vi "ImPro - Sharpen.vi"(8 "error in (no error)":errorcluster, 10 "24-bit pixmap In":u32[][](array[numeric]), 11 "Sharpen?":bool) -> (0 "error out":errorcluster, 2 "24-bit pixmap Out":u32[][](array[numeric]))   [LabVIEW 2023]
panel:
  in  "Scaling Factor":dbl=5.0 min=0.0
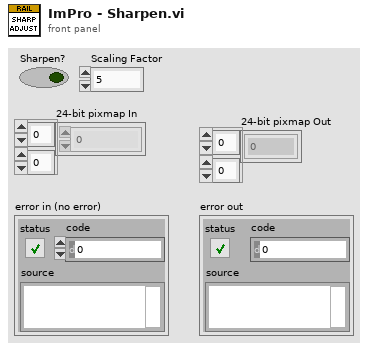
[diagram p1: front panel]
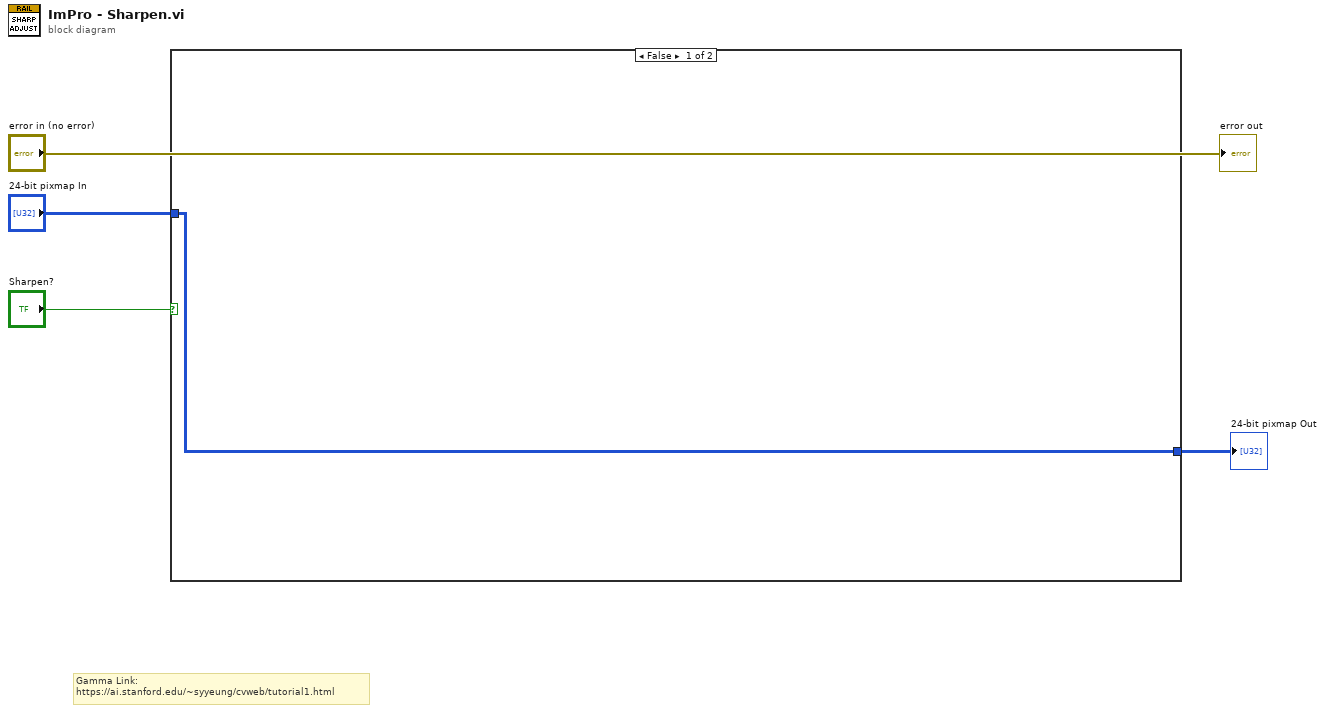
[diagram p0: block diagram]
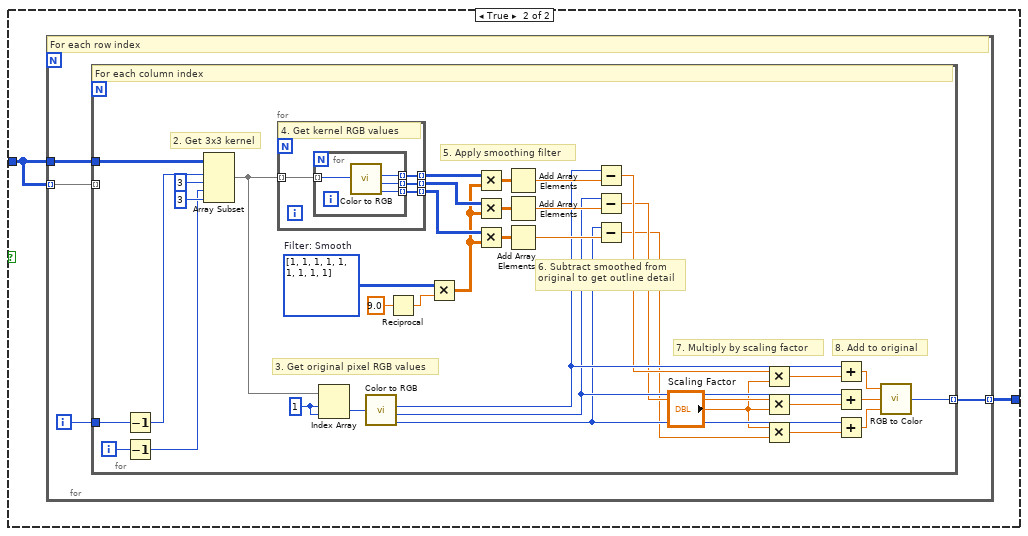
[diagram p2: hidden frame]
diagram:
  # "Gamma Link:\nhttps://ai.stanford.edu/~syyeung/cvweb/tutorial1.html"
  n1 = case shown="False" "Sharpen?" {
    tunnel: "24-bit pixmap In" -> [w5 w7]
    tunnel: [w5 w6] -> w2
    frame False {
    }
    frame True {
      n2 = for {
        tunnel: w7 -> [w11] mode=indexing
        tunnel: w7 -> [w10]
        tunnel: [w8] -> w6 mode=indexing
        i -> [w9]
        # "For each row index"
        n3 = for {
          tunnel: w11 -> [_] mode=indexing
          tunnel: w9 -> [w45]
          tunnel: w10 -> [w47]
          tunnel: [w35] -> w8 mode=indexing
          i -> [w44]
          w29 = 1 ("index (row)")
          w33 = i32[][] [[1, 1, 1], [1, 1, 1], [1, 1, 1]]  # Filter: Smooth
          # "8. Add to original"
          # "7. Multiply by scaling factor"
          # "6. Subtract smoothed from\noriginal to get outline detail"
          # "5. Apply smoothing filter"
          # "3. Get original pixel RGB values"
          # "2. Get 3x3 kernel"
          # "For each column index"
          n4 = Decrement(x=w45) -> (x-1=w43:i32)
          n5 = Decrement(x=w44) -> (x-1=w42:i32)
          n6 = Array Subset(array=w47, index (row)=w43, length (row)=3 ("length"), index (col)=w42, length (col)=3 ("length")) -> (w30:u32[][])
          n7 = for {
            tunnel: w30 -> [w52] mode=indexing
            tunnel: [w51] -> w40 mode=indexing
            tunnel: [w50] -> w37 mode=indexing
            tunnel: [w49] -> w36 mode=indexing
            # "4. Get kernel RGB values"
            n8 = for {
              tunnel: w52 -> [w56] mode=indexing
              tunnel: [w55] -> w51 mode=indexing
              tunnel: [w54] -> w50 mode=indexing
              tunnel: [w53] -> w49 mode=indexing
              n9 = call <vilib>:"Color to RGB.vi"("Color"=w56) -> ("R"=w55:u8, "G"=w54:u8, "B"=w53:u8)  [unwired: 1 out]
            }
          }
          n10 = Index Array(array=w30, index (row)=w29, index (col)=w29) -> (element=w28:u32)
          n11 = call <vilib>:"Color to RGB.vi"("Color"=w28) -> ("R"=w24:u8, "G"=w23:u8, "B"=w22:u8)  [unwired: 1 out]
          n12 = Reciprocal(x=9.0) -> (1/x=w34:dbl)
          n13 = Multiply(x=w33, y=w34) -> (x*y=w31:dbl[][])
          n14 = Multiply(x=w40, y=w31) -> (x*y=w41:dbl[][])
          n15 = Multiply(x=w37, y=w31) -> (x*y=w39:dbl[][])
          n16 = Multiply(x=w36, y=w31) -> (x*y=w38:dbl[][])
          n17 = Add Array Elements(numeric array=w41) -> (sum=w27:dbl)
          n18 = Add Array Elements(numeric array=w39) -> (sum=w25:dbl)
          n19 = Add Array Elements(numeric array=w38) -> (sum=w26:dbl)
          n20 = Subtract(x=w24, y=w27) -> (x-y=w17:dbl)
          n21 = Subtract(x=w23, y=w25) -> (x-y=w16:dbl)
          n22 = Subtract(x=w22, y=w26) -> (x-y=w13:dbl)
          n23 = Multiply(x=w17, y="Scaling Factor") -> (x*y=w18:dbl)
          n24 = Multiply(x=w16, y="Scaling Factor") -> (x*y=w15:dbl)
          n25 = Multiply(x="Scaling Factor", y=w13) -> (x*y=w14:dbl)
          n26 = Add(x=w24, y=w18) -> (x+y=w21:dbl)
          n27 = Add(x=w23, y=w15) -> (x+y=w20:dbl)
          n28 = Add(x=w22, y=w14) -> (x+y=w19:dbl)
          n29 = call <vilib>:"RGB to Color.vi"("B"=w19, "G"=w20, "R"=w21) -> ("Color"=w35:u32)
        }
      }
    }
  }
  "24-bit pixmap Out" <- w2
  "error out" <- "error in (no error)"
